vi "GetEventInterface.vi"(8 "error in (no error)":errorcluster, 11 "Engine in":refnum<class "Engine.lvclass">) -> (0 "error out":errorcluster, 2 "Event Interface":refnum<class "EngineEventInterface.lvclass">, 3 "Engine out":refnum<class "Engine.lvclass">)   [LabVIEW 2020, in "GLF.lvlib" / "Engine.lvclass"]
uses:
  Engine.lvclass
  Engine.lvclass/Engine.ctl
  EngineEventInterface/EngineEventInterface.lvclass
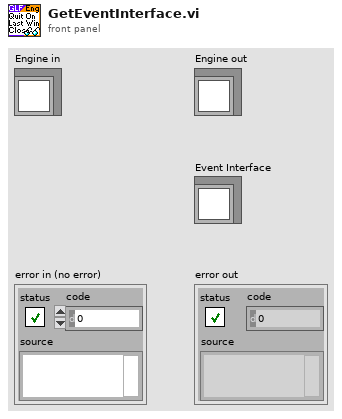
[diagram p1: front panel]
types:
  T1 = typedef "GLF.lvlib/Engine.lvclass/DVR--cluster.ctl" = cluster{"CMD Queue":T2, "Config":T3, "Ctxt":T5, "Metrics":T6, "Debug":T7, "ID To Window":map{T9, refnum<class "Window.lvclass">}, "Window To Handle":map{refnum<class "Window.lvclass">, i64}, "Event Interface":refnum<class "EngineEventInterface.lvclass">}
  T2 = typedef "GLF.lvlib/Engine.lvclass/Command--queue.ctl" = refnum<queue>
  T3 = typedef "GLF.lvlib/Engine.lvclass/Config--cluster.ctl" = cluster{"Quit On Last Window Closed":bool, "VSync":T4, "FPS Target":dbl}
  T4 = typedef "GLF.lvlib/Engine.lvclass/VSync--enum.ctl" = enum16{"Disabled", "Enabled", "Adaptative"}
  T5 = typedef "GLF.lvlib/Engine.lvclass/Context--cluster.ctl" = cluster{"VSync Enabled":bool}
  T6 = typedef "GLF.lvlib/Engine.lvclass/Metrics--cluster.ctl" = cluster{"Uptime [ms]":u64, "Loop Time [ms]":u64, "Timer [ns]":u64, "Poll Events [ns]":u64, "Dequeue CMD [ns]":u64, "Update Layout [ns]":u64, "Render [ns]":u64}
  T7 = typedef "GLF.lvlib/Engine.lvclass/Debug--cluster.ctl" = cluster{"Unhandled Events":map{T8, u64}}
  T8 = typedef "SDL3.lvlib/Events.lvlib/EventType--enum.ctl" = enum16{"LV_NONE", "LV_UNSUPPORTED", "SDL_EVENT_QUIT", "SDL_EVENT_LOCALE_CHANGED", "SDL_EVENT_SYSTEM_THEME_CHANGED", "SDL_EVENT_DISPLAY_ORIENTATION", "SDL_EVENT_DISPLAY_ADDED", "SDL_EVENT_DISPLAY_REMOVED", "SDL_EVENT_DISPLAY_MOVED", "SDL_EVENT_DISPLAY_DESKTOP_MODE_CHANGED", "SDL_EVENT_DISPLAY_CURRENT_MODE_CHANGED", "SDL_EVENT_DISPLAY_CONTENT_SCALE_CHANGED", "SDL_EVENT_WINDOW_SHOWN", "SDL_EVENT_WINDOW_HIDDEN", "SDL_EVENT_WINDOW_EXPOSED", "SDL_EVENT_WINDOW_MOVED", "SDL_EVENT_WINDOW_RESIZED", "SDL_EVENT_WINDOW_PIXEL_SIZE_CHANGED", "SDL_EVENT_WINDOW_METAL_VIEW_RESIZED", "SDL_EVENT_WINDOW_MINIMIZED", "SDL_EVENT_WINDOW_MAXIMIZED", "SDL_EVENT_WINDOW_RESTORED", "SDL_EVENT_WINDOW_MOUSE_ENTER", "SDL_EVENT_WINDOW_MOUSE_LEAVE", "SDL_EVENT_WINDOW_FOCUS_GAINED", "SDL_EVENT_WINDOW_FOCUS_LOST", "SDL_EVENT_WINDOW_CLOSE_REQUESTED", "SDL_EVENT_WINDOW_HIT_TEST", "SDL_EVENT_WINDOW_ICCPROF_CHANGED", "SDL_EVENT_WINDOW_DISPLAY_CHANGED", "SDL_EVENT_WINDOW_DISPLAY_SCALE_CHANGED", "SDL_EVENT_WINDOW_SAFE_AREA_CHANGED", "SDL_EVENT_WINDOW_OCCLUDED", "SDL_EVENT_WINDOW_ENTER_FULLSCREEN", "SDL_EVENT_WINDOW_LEAVE_FULLSCREEN", "SDL_EVENT_WINDOW_DESTROYED", "SDL_EVENT_WINDOW_HDR_STATE_CHANGED", "SDL_EVENT_KEY_DOWN", "SDL_EVENT_KEY_UP", "SDL_EVENT_TEXT_EDITING", "SDL_EVENT_TEXT_INPUT", "SDL_EVENT_KEYMAP_CHANGED", "SDL_EVENT_KEYBOARD_ADDED", "SDL_EVENT_KEYBOARD_REMOVED", "SDL_EVENT_TEXT_EDITING_CANDIDATES", "SDL_EVENT_MOUSE_MOTION", "SDL_EVENT_MOUSE_BUTTON_DOWN", "SDL_EVENT_MOUSE_BUTTON_UP", "SDL_EVENT_MOUSE_WHEEL", "SDL_EVENT_MOUSE_ADDED", "SDL_EVENT_MOUSE_REMOVED", "SDL_EVENT_JOYSTICK_AXIS_MOTION", "SDL_EVENT_JOYSTICK_BALL_MOTION", "SDL_EVENT_JOYSTICK_HAT_MOTION", "SDL_EVENT_JOYSTICK_BUTTON_DOWN", "SDL_EVENT_JOYSTICK_BUTTON_UP", "SDL_EVENT_JOYSTICK_ADDED", "SDL_EVENT_JOYSTICK_REMOVED", "SDL_EVENT_JOYSTICK_BATTERY_UPDATED", "SDL_EVENT_JOYSTICK_UPDATE_COMPLETE", "SDL_EVENT_GAMEPAD_AXIS_MOTION", "SDL_EVENT_GAMEPAD_BUTTON_DOWN", "SDL_EVENT_GAMEPAD_BUTTON_UP", "SDL_EVENT_GAMEPAD_ADDED", "SDL_EVENT_GAMEPAD_REMOVED", "SDL_EVENT_GAMEPAD_REMAPPED", "SDL_EVENT_GAMEPAD_TOUCHPAD_DOWN", "SDL_EVENT_GAMEPAD_TOUCHPAD_MOTION", "SDL_EVENT_GAMEPAD_TOUCHPAD_UP", "SDL_EVENT_GAMEPAD_SENSOR_UPDATE", "SDL_EVENT_GAMEPAD_UPDATE_COMPLETE", "SDL_EVENT_GAMEPAD_STEAM_HANDLE_UPDATED", "SDL_EVENT_FINGER_DOWN", "SDL_EVENT_FINGER_UP", "SDL_EVENT_FINGER_MOTION", "SDL_EVENT_CLIPBOARD_UPDATE", "SDL_EVENT_DROP_FILE", "SDL_EVENT_DROP_TEXT", "SDL_EVENT_DROP_BEGIN", "SDL_EVENT_DROP_COMPLETE", "SDL_EVENT_DROP_POSITION", "SDL_EVENT_AUDIO_DEVICE_ADDED", "SDL_EVENT_AUDIO_DEVICE_REMOVED", "SDL_EVENT_AUDIO_DEVICE_FORMAT_CHANGED", "SDL_EVENT_SENSOR_UPDATE", "SDL_EVENT_PEN_PROXIMITY_IN", "SDL_EVENT_PEN_PROXIMITY_OUT", "SDL_EVENT_PEN_DOWN", "SDL_EVENT_PEN_UP", "SDL_EVENT_PEN_BUTTON_DOWN", "SDL_EVENT_PEN_BUTTON_UP", "SDL_EVENT_PEN_MOTION", "SDL_EVENT_PEN_AXIS", "SDL_EVENT_CAMERA_DEVICE_ADDED", "SDL_EVENT_CAMERA_DEVICE_REMOVED", "SDL_EVENT_CAMERA_DEVICE_APPROVED", "SDL_EVENT_CAMERA_DEVICE_DENIED", "SDL_EVENT_RENDER_TARGETS_RESET", "SDL_EVENT_RENDER_DEVICE_RESET", "SDL_EVENT_POLL_SENTINEL", "SDL_EVENT_USER"}
  T9 = typedef "SDL3.lvlib/Video.lvlib/WindowID--integer.ctl" = u32
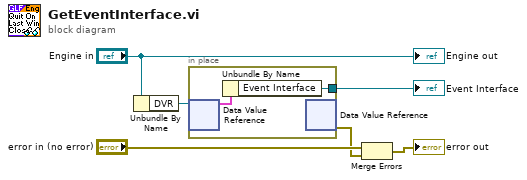
[diagram p0: block diagram]
diagram:
  n1 = Unbundle By Name("Engine in") -> ("DVR"=w3:refnum<data-value>)
  n2 = in-place {
    in-place-border: [w8] -> w1
    n3 = in-place-dvr #1(w3) -> (w7:T1)  [unwired: 1 out]
    n4 = Unbundle By Name(w7) -> ("Event Interface"=w8:refnum<class "EngineEventInterface.lvclass">)
    n5 = in-place-dvr #1() -> (w2:errorcluster)  [unwired: 1 in, 1 out]
  }
  "Event Interface" <- w1
  n6 = Merge Errors("error in (no error)", w2) -> (→"error out":errorcluster)
  "Engine out" <- "Engine in"
